vi "Close Reference.vi"(8 "error in (no error)":errorcluster, 11 "HTTP GET Async handle":T1) -> (0 "error out":errorcluster)   [LabVIEW 2019, in "HTTP Client Extensions.lvlib" / "Get Async.lvlib"]
uses:
  Get Async.lvlib
  GET Async.lvclass
  controls/Refnum Type - Enum.ctl
  controls/Refnum Type.ctl
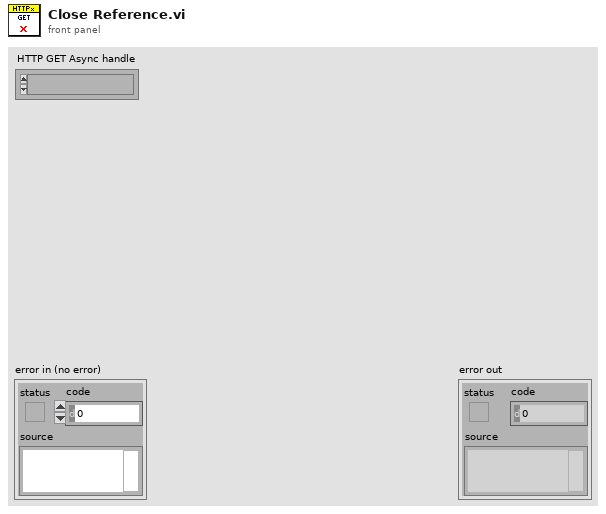
[diagram p1: front panel]
types:
  T1 = typedef "HTTP Client Extensions.lvlib/Get Async.lvlib/Refnum Type.ctl" = refnum<k1>
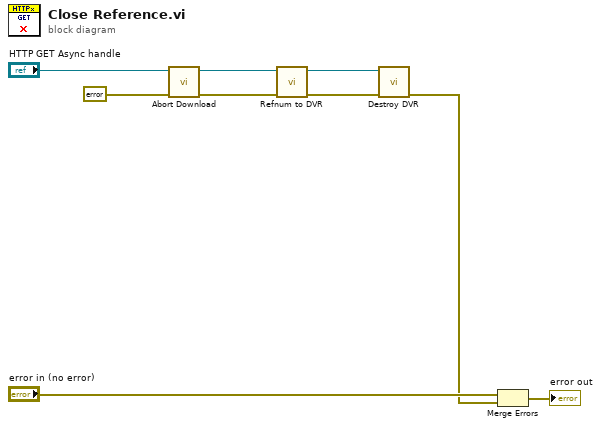
[diagram p0: block diagram]
diagram:
  n1 = call "Abort Download.vi"("error in (no error)"=errorcluster {"status"=FALSE, "code"=0, "source"=""}, "HTTP GET Async handle"="HTTP GET Async handle") -> ("error out"=w5:errorcluster, "HTTP GET Async handle out"=w2:T1)  [unwired: 8 in]
  n2 = call "Refnum to DVR.vi"("Refnum out"=w2) -> ("Data Value Reference in"=w1:refnum<data-value>)  [unwired: 10 in]
  n3 = call "Destroy DVR.vi"("error in (no error)"=w5, "HTTP GET Async ref in"=w1) -> ("error out"=w4:errorcluster)  [unwired: 9 in]
  n4 = Merge Errors("error in (no error)", w4) -> (→"error out":errorcluster)
